vi "duf file read.vi"(8 "error in (no error)":errorcluster, 11 "Main Ref":T1) -> (0 "error out":errorcluster, 3 "Main Ref 2":T1)   [LabVIEW 2025]
panel:
  in  "Fuel Description :":string
  in  "Batch Ref Number :":string
  in  "Date and Time :":string
  out "text":string
  out "Tested Date":string
  out "Tested By :-":string
  out "Operator :":string
  out "XY Graph":cluster{"X":dbl[], "Y":dbl[]}[](graph)
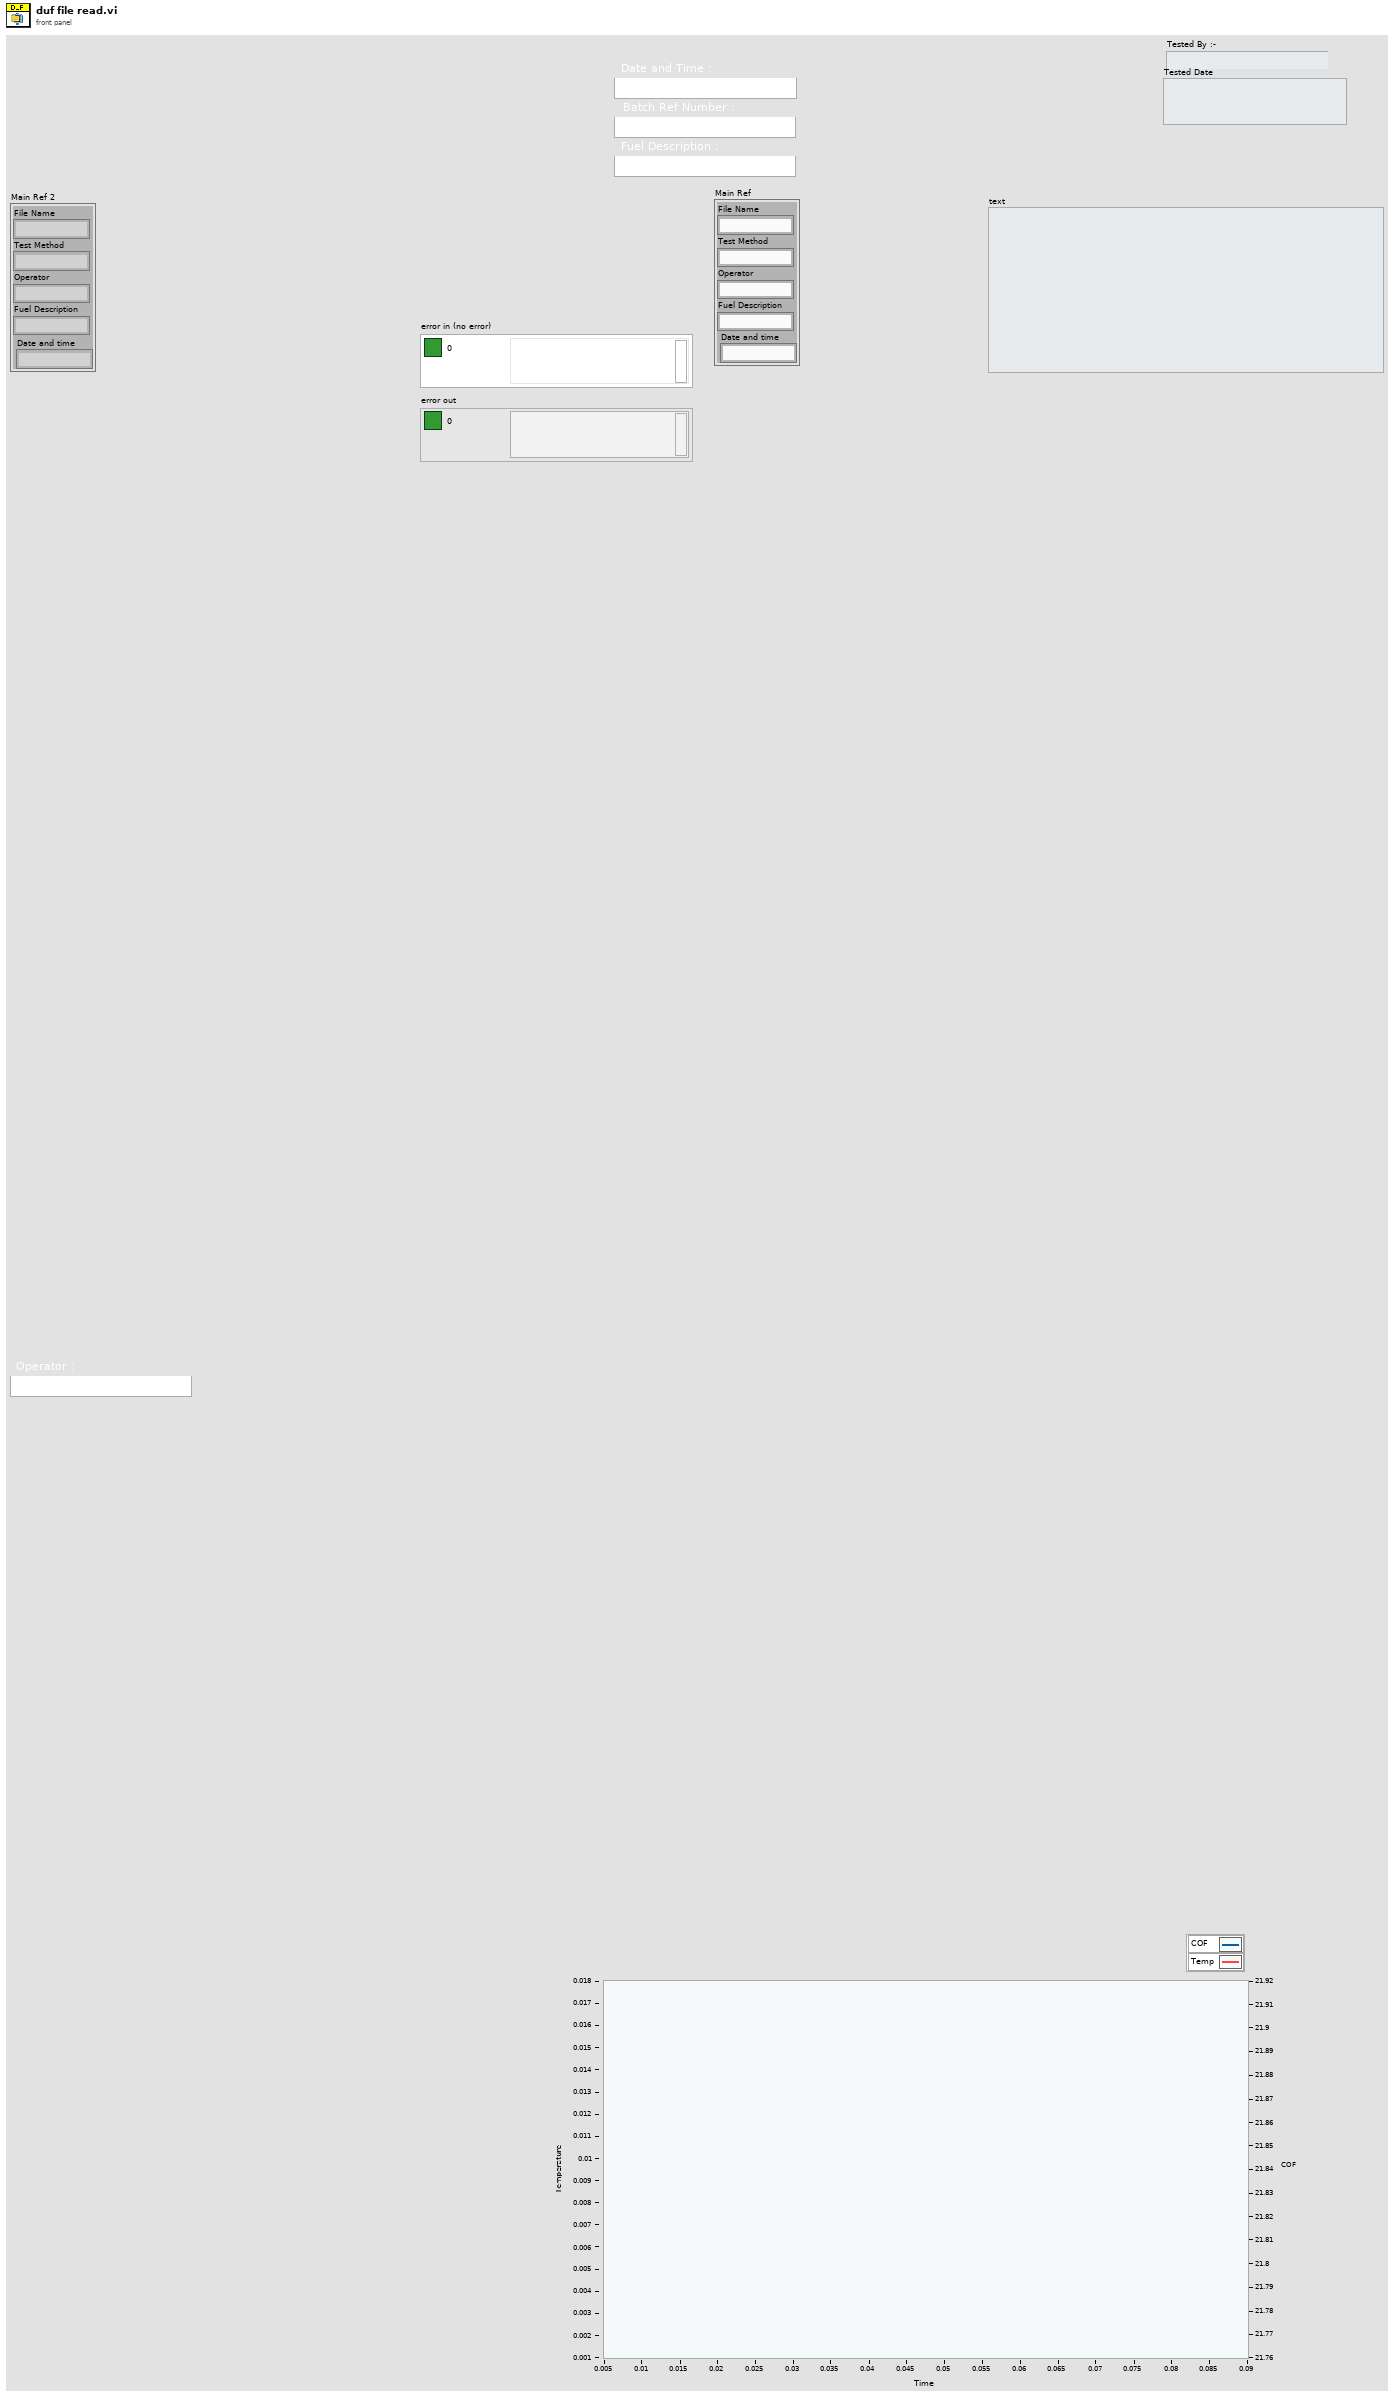
[diagram p1: front panel]
types:
  T1 = cluster{"File Name":string, "Test Method":string, "Operator":string, "Fuel Description":string, "Date and time":string}
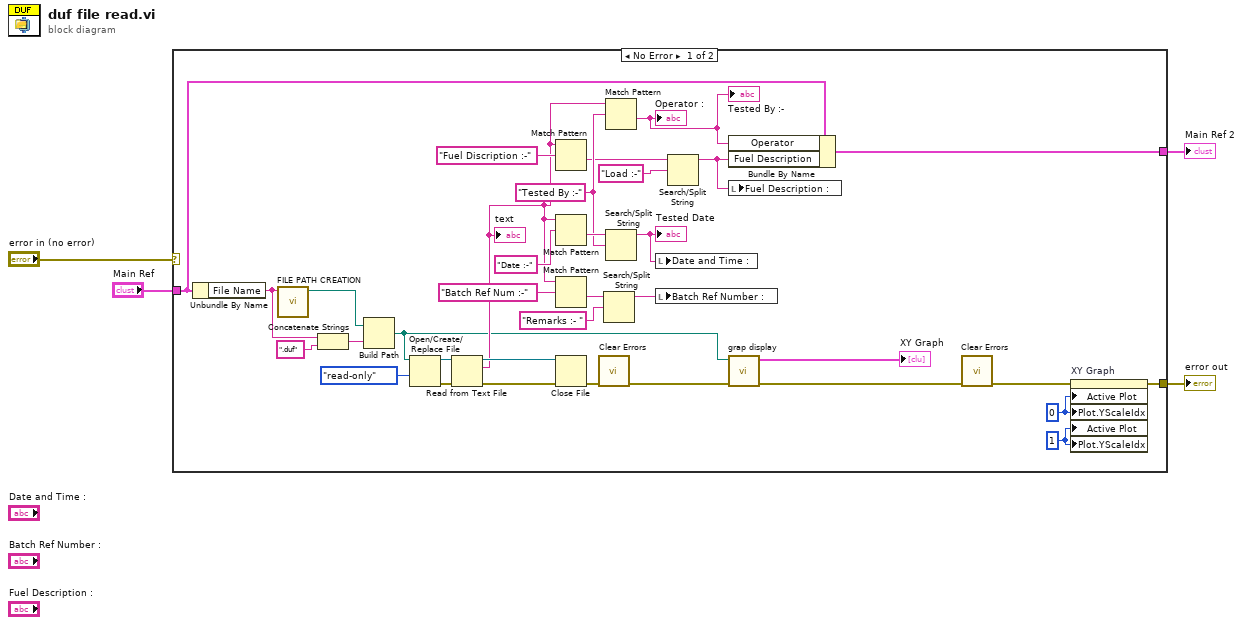
[diagram p0: block diagram]
diagram:
  n1 = case shown="No Error" "error in (no error)" {
    tunnel: "Main Ref" -> [w6 w39]
    tunnel: [w9 _] -> w3
    tunnel: [w5 w39] -> w1
    frame No Error {
      w25 = u32 1 ("Active Plot")
      w26 = u32 0 ("Active Plot")
      w31 = "Tested By :-" ("regular expression")
      n2 = Unbundle By Name(w6) -> ("File Name"=w11:string)
      n3 = call "FILE PATH CREATION.vi"("FILE NAME :"=w11) -> ("FILE OUT"=w13:path)  [unwired: 9 in, 1 out]
      n4 = Concatenate Strings(w11, ".duf" ("Substring")) -> (w14:string)
      n5 = Build Path(base path=w13, name or relative path=w14) -> (appended path=w10:path)
      n6 = Open/Create/Replace File(file path (use dialog)=w10, access (0:read/write)=enum16{"read/write", "read-only", "write-only"}."read-only") -> (refnum out=w36:refnum<file>, error out=w37:errorcluster)  [unwired: 4 in, 1 out]
      n7 = Read from Text File(file (use dialog)=w36, error in=w37) -> (refnum out=w34:refnum<file>, text=w16:string, error out=w35:errorcluster)  [unwired: 2 in, 1 out]
      "text" <- w16
      n8 = Match Pattern(string=w16, regular expression="Fuel Discription :-") -> (after substring=w18:string)  [unwired: 1 in, 3 out]
      n9 = Match Pattern(string=w16, regular expression="Date :-") -> (after substring=w32:string)  [unwired: 1 in, 3 out]
      n10 = Match Pattern(string=w16, regular expression="Batch Ref Num :-") -> (after substring=w20:string)  [unwired: 1 in, 3 out]
      n11 = Close File(refnum=w34, error in=w35) -> (error out=w24:errorcluster)  [unwired: 1 out]
      n12 = call <vilib>:"Clear Errors.vi"("error in (no error)"=w24) -> ("error out"=w23:errorcluster)  [unwired: 5 in, 1 out]
      n13 = Search/Split String(string=w20, search string/char (-)="Remarks :- ") -> (substring before match=w15:string)  [unwired: 1 in, 2 out]
      n14 = Match Pattern(string=w16, regular expression=w31) -> (after substring=w8:string)  [unwired: 1 in, 3 out]
      "Tested By :-" <- w8
      "Operator :" <- w8
      n15 = Search/Split String(string=w32, search string/char (-)=w31) -> (substring before match=w30:string)  [unwired: 1 in, 2 out]
      "Tested Date" <- w30
      n16 = local write "Date and Time :"(w30) -> ()
      n17 = local write "Batch Ref Number :"(w15) -> ()
      n18 = Search/Split String(string=w18, search string/char (-)="Load :-") -> (substring before match=w7:string)  [unwired: 1 in, 2 out]
      n19 = Bundle By Name(cluster=w6, "Operator"=w8, "Fuel Description"=w7) -> (w5:T1)
      n20 = local write "Fuel Description :"(w7) -> ()
      n21 = call "grap display.vi"("error in"=w23, "file path (dialog if empty)"=w10) -> ("error out"=w28:errorcluster, "XY GRAPH"=→"XY Graph":cluster{"X":dbl[], "Y":dbl[]}[])  [unwired: 8 in]
      n22 = call <vilib>:"Clear Errors.vi"("error in (no error)"=w28) -> ("error out"=w27:errorcluster)  [unwired: 5 in, 1 out]
      n23 = property on="XY Graph" class="XYGraph (strict)"(error in=w27, "Active Plot"=w26, "Plot.YScaleIdx"=w26, "Active Plot"=w25, "Plot.YScaleIdx"=w25) -> (error out=w9:errorcluster)  [unwired: 1 in, 1 out]
    }
    frame Error {
    }
  }
  "error out" <- w3
  "Main Ref 2" <- w1
